vi "Vision Processing Jims way.vi"(0 "Image In":T2, 7 "error in":errorcluster) -> (20 "Image Out":T2, 21 "Matches (Pattern Matching 1)":T1(array[cluster]) {"Bounding Box"."y" format="%.2f"; "Bounding Box"."x" format="%.2f"; "Position"."y" format="%.2f"; "Position"."x" format="%.2f"; "Score" format="%.2f"; "Scale" format="%.2f"; "Angle" format="%.2f"}, 22 "Calibrated Matches (Pattern Matching 1)":T1(array[cluster]) {"Bounding Box"."y" format="%.2f"; "Bounding Box"."x" format="%.2f"; "Position"."y" format="%.2f"; "Position"."x" format="%.2f"; "Score" format="%.2f"; "Scale" format="%.2f"; "Angle" format="%.2f"}, 23 "Number of Matches (Pattern Matching 1)":i32, 27 "error out":errorcluster)   [LabVIEW 2018]
uses:
  <vilib>/vision/Image Controls.llb/IMAQ Image.ctl
  <vilib>/vision/Pattern Matching.llb/IMAQ Pattern Match Advanced Options.ctl
  <vilib>/vision/NI_Vision_Development_Module.lvlib
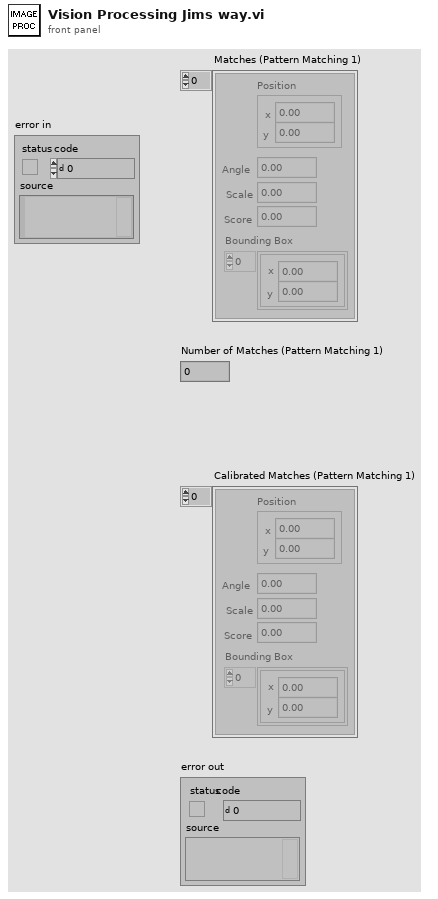
[diagram p1: front panel]
types:
  T1 = cluster{"Position":cluster{"x":sgl, "y":sgl}, "Angle":sgl, "Scale":sgl, "Score":sgl, "Bounding Box":cluster{"x":sgl, "y":sgl}[]}[]
  T2 = typedef "IMAQ Image.ctl" = refnum<image>
  T3 = typedef "IMAQ Pattern Match Advanced Options.ctl" = u16
  T4 = cluster{"Number of Matches Requested":i32, "Minimum Match Score":sgl, "Angle Ranges":cluster{"Start Angle":sgl, "End Angle":sgl}[]}
  T5 = cluster{"Global Rectangle":i32[], "Contours":cluster{"ID":enum32{"External", "Internal"}, "Type":u32, "Coordinates":i32[]}[]}
  T6 = cluster{"Brightness":sgl, "Contrast":sgl, "Gamma":sgl}
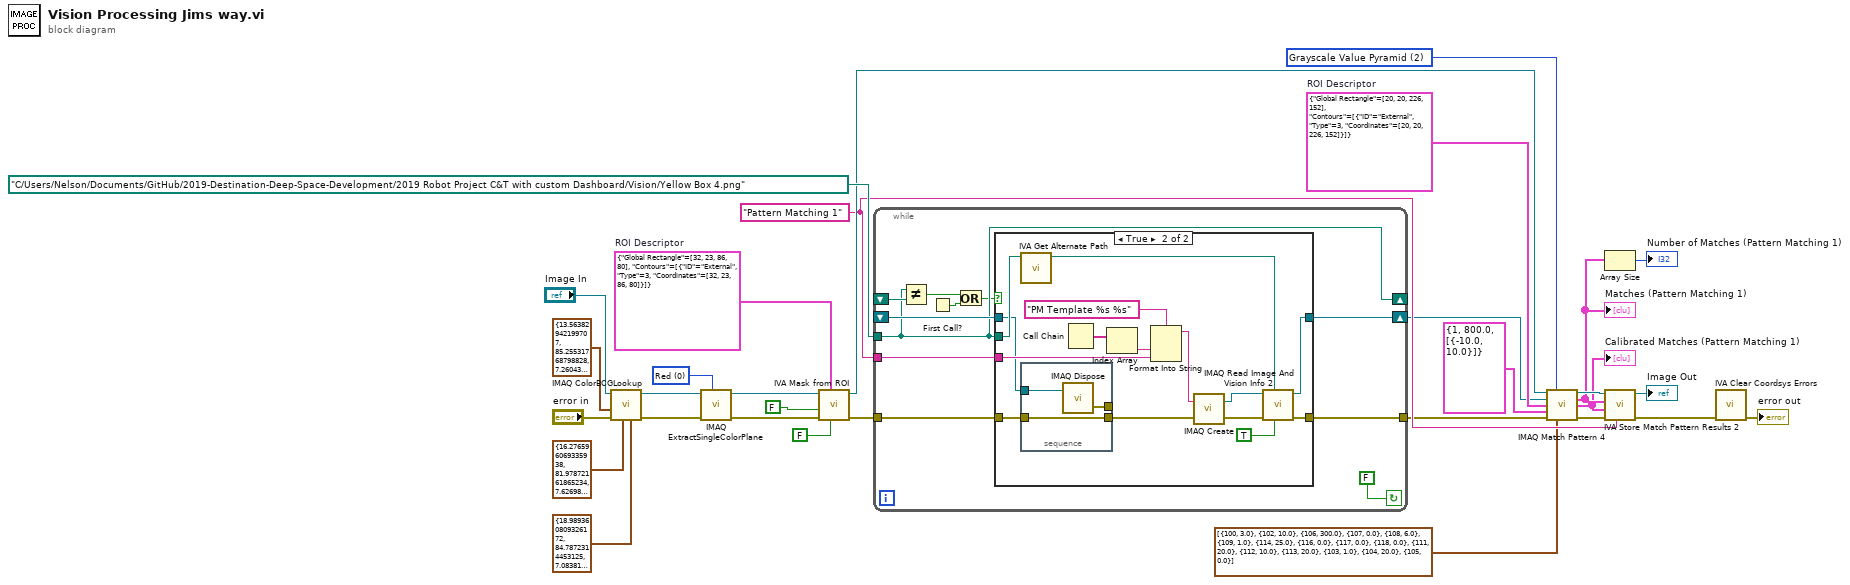
[diagram p0: block diagram]
diagram:
  w12 = 2 items=["All", "Low Discrepancy Sampling", "Grayscale Value Pyramid", "Gradients Pyramid"] ("Algorithm")
  w8 = "Pattern Matching 1" ("Step Name")
  w11 = T5 {"Global Rectangle"=[20, 20, 226, 152], "Contours"=[{"ID"=enum."External", "Type"=3, "Coordinates"=[20, 20, 226, 152]}]}  # ROI Descriptor
  w23 = T5 {"Global Rectangle"=[32, 23, 86, 80], "Contours"=[{"ID"=enum."External", "Type"=3, "Coordinates"=[32, 23, 86, 80]}]}  # ROI Descriptor
  w26 = 0 items=["Red", "Green", "Blue", "Hue", "Saturation", "Luminance", "Value", "Intensity"] ("Color Plane")
  n1 = call "IMAQ ColorBCGLookup"("Blue BCG Values"=T6 {"Brightness"=18.98936, "Contrast"=84.78723, "Gamma"=7.083818}, "Green BCG Values"=T6 {"Brightness"=16.276596, "Contrast"=81.97872, "Gamma"=7.626986}, "error in (no error)"="error in", "Red BCG Values"=T6 {"Brightness"=13.563829, "Contrast"=85.25532, "Gamma"=7.2604337}, "Image Src"="Image In") -> ("error out"=w24:errorcluster, "Image Dst Out"=w25:T2)  [unwired: 2 in, 3 out]
  n2 = call "IMAQ ExtractSingleColorPlane"("Color Plane"=w26, "error in (no error)"=w24, "Image Src"=w25) -> ("error out"=w19:errorcluster, "Image Dst Out"=w21:T2)  [unwired: 1 in, 6 out]
  n3 = call <vilib>:"IVA Mask from ROI.vi"("Shrink"=FALSE, "ROI Descriptor"=w23, "error in (no error)"=w19, "Out / In"=FALSE, "Image Src"=w21) -> ("error out"=w13:errorcluster, "Image Out"=w17:T2)  [unwired: 5 out]
  n4 = while {
    shift-right: [w42] -> w5
    shift-left: _ -> [w41]
    tunnel: [w39] -> w4
    tunnel: w13 -> [w38]
    tunnel: path "C:/Users/Nelson/Documents/GitHub/2019-Destination-Deep-Space-Development/2019 Robot Project C&T with custom Dashboard/Vision/Yellow Box 4.png" ("Template File Path") -> [w35]
    tunnel: w8 -> [w37]
    shift-right: [w35] -> _
    shift-left: _ -> [w36]
    stop <- FALSE continue-if-true
    n5 = Not Equal?(x=w35, y=w36) -> (x != y?=w33:bool)
    n6 = First Call?() -> (First Call?: T/F=w34:bool)
    n7 = Or(x=w33, y=w34) -> (x .or. y?=w32:bool)
    n8 = case shown="True" w32 {
      tunnel: [w44 w49] -> w42
      tunnel: w41 -> [w44 w53]
      tunnel: [w43 w50] -> w39
      tunnel: w38 -> [w43 w52]
      tunnel: w35 -> [_ w54]
      tunnel: w37 -> [_ w55]
      frame False {
      }
      frame True {
        n9 = call <vilib>:"IVA Get Alternate Path.vi"("Path In"=w54) -> ("Path Out"=w51:path)  [unwired: 10 out]
        n10 = stacked-sequence {
          tunnel: w53 -> [w62]
          tunnel: w52 -> [w61]
          tunnel: [w61] -> w46
          tunnel: [w60] -> _
          frame #0 {
            n11 = call "IMAQ Dispose"("Image"=w62) -> ("error out"=w60:errorcluster)  [unwired: 2 in, 3 out]
          }
        }
        n12 = Call Chain() -> (call chain=w57:string[])
        n13 = Index Array(array=w57) -> (element=w56:string)  [unwired: 1 in]
        n14 = Format Into String(format string="PM Template %s %s" ("Image Name"), w56, w55) -> (resulting string=w59:string)  [unwired: 2 in, 1 out]
        n15 = call "IMAQ Create"("Image Name"=w59, "error in (no error)"=w46) -> ("New Image"=w48:T2, "error out"=w47:errorcluster)  [unwired: 2 in, 1 out]
        n16 = call "IMAQ Read Image And Vision Info 2"("Use File Path Image Type"=TRUE, "File Path"=w51, "error in (no error)"=w47, "Image"=w48) -> ("error out"=w50:errorcluster, "Image Out"=w49:T2)  [unwired: 5 in, 1 out]
      }
    }
  }
  n17 = call "IMAQ Match Pattern 4"("Image"=w17, "Algorithm"=w12, "Template Image"=w5, "ROI Descriptor"=w11, "Parameters"=T4 {"Number of Matches Requested"=1, "Minimum Match Score"=800.0, "Angle Ranges"=[{"Start Angle"=-10.0, "End Angle"=10.0}]}, "error in (no error)"=w4, "Advanced Options"=cluster{"Item":T3, "Value":dbl}[] [{"Item"=100, "Value"=3.0}, {"Item"=102, "Value"=10.0}, {"Item"=106, "Value"=300.0}, {"Item"=107, "Value"=0.0}, {"Item"=108, "Value"=6.0}, {"Item"=109, "Value"=1.0}, {"Item"=114, "Value"=25.0}, {"Item"=116, "Value"=0.0}, {"Item"=117, "Value"=0.0}, {"Item"=118, "Value"=0.0}, {"Item"=111, "Value"=20.0}, {"Item"=112, "Value"=10.0}, {"Item"=113, "Value"=20.0}, {"Item"=103, "Value"=1.0}, {"Item"=104, "Value"=20.0}, {"Item"=105, "Value"=0.0}]) -> ("Image (duplicate)"=w14:T2, "Matches (pixel)"=w7:T1, "Matches (real-world)"=w6:T1, "error out"=w15:errorcluster)  [unwired: 4 in, 1 out]
  "Matches (Pattern Matching 1)" <- w7
  "Calibrated Matches (Pattern Matching 1)" <- w6
  n18 = Array Size(array=w7) -> (size(s)=→"Number of Matches (Pattern Matching 1)":i32)
  n19 = call <vilib>:"IVA Store Match Pattern Results 2.vi"("Step Name"=w8, "error in (no error)"=w15, "Matches (real-world)"=w6, "Matches (pixel)"=w7, "Image in"=w14) -> ("error out"=w3:errorcluster, "Image dup"=→"Image Out":T2)  [unwired: 1 in, 4 out]
  n20 = call <vilib>:"IVA Clear Coordsys Errors.vi"("error in (no error)"=w3) -> ("error out"=→"error out":errorcluster)  [unwired: 10 in]
